vi "main.vi"() -> ()   [LabVIEW 2018]
uses:
  <vilib>/NI/Modbus Library/API/Wrapper/Create TCP Slave.vi
  <vilib>/NI/Modbus Library/API/Slave/Modbus Slave.lvclass
  <vilib>/NI/Modbus Library/API/Wrapper/API Main.lvlib
panel:
  in  "x+1":i32
  in  "擦除曲线":bool
  in  "PC启动信号":bool
  in  "PC就绪":bool
  out "远程/本地控制布尔":bool
  out "XY图":cluster{i32[], sgl[]}[](graph)
  in  "远程/本地控制":bool
  out "远程/本地控制标题":string="远程/本地"
  out "当前档位":string="当前档位"
  in  "档位目标内容":string
  out "PCTOUTAC的当前档位":string="PCTOUTAC的当前档位"
  out "档位目标内容远程":string
  in  "档位目标内容本地":string
  out "档位目标":string="配方编号"
  out "UTACTOPC的目标档位":string="UTACTOPC的配方编号"
  in  "中英文":string(combo)
  in  "编辑设定参数":bool
  in  "编辑配方":bool
  in  "退出":bool
  out "设置":string="设置"
  in  "PC换挡不成功":bool
  in  "PC换挡到位":bool
  in  "PC正在换挡":bool
  in  "PC急停":bool
  in  "PC学习":bool
  in  "PC故障":bool
  in  "PC运行/停机":bool
  out "PCOUTAC的DI信号":string="PCTOUTAC的DI信号"
  in  "UTAC复位到原点":bool
  in  "UTAC故障复位":bool
  in  "UTAC急停":bool
  in  "UTAC故障":bool
  in  "UTAC运行/停机":bool
  out "UTACTOPC的DO信号":string="UTACTOPC的DO信号"
  in  "设置":bool
  in  "总测试次数文本":string
  in  "动作数量文本":string
  in  "备注文本":string
  in  "样品编号文本":string
  in  "零件编号文本":string
  in  "零件名称文本":string
  in  "项目编号文本":string
  out "总测试次数":string="总测试次数"
  out "动作数量":string="动作数量"
  out "备注":string="备注"
  out "样品编号":string="样品编号"
  out "零件编号":string="零件编号"
  out "零件名称":string="零件名称"
  out "项目编号":string="项目编号"
  out "项目信息":string="项目信息"
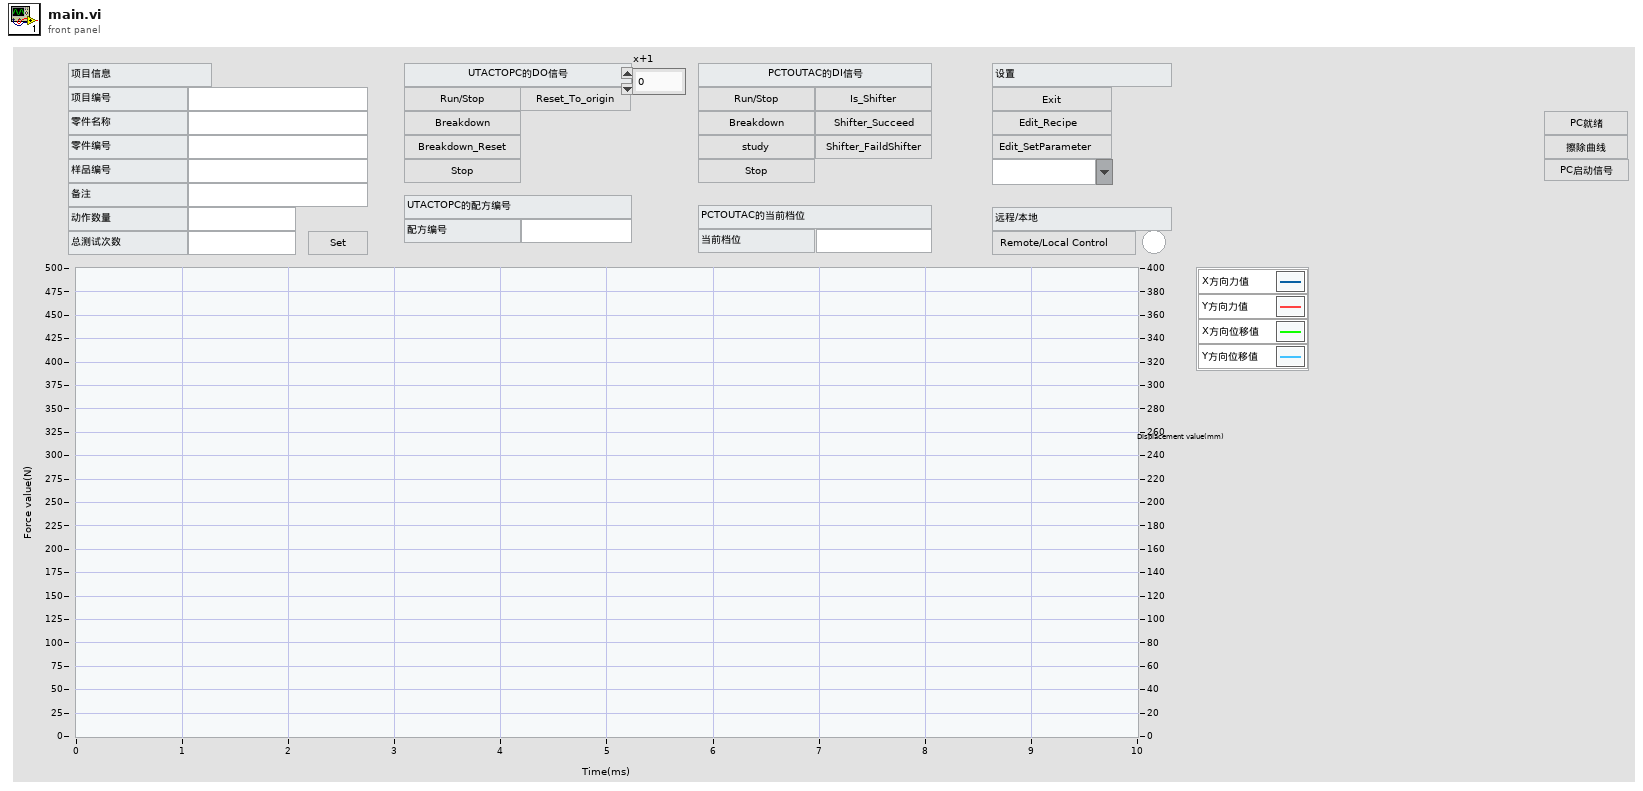
[diagram p1: front panel]
types:
  T1 = cluster{"主站IP":u32, "组号":u8, "帧号":u16, "时间戳":u64}
  T2 = cluster{"X方向力值":sgl, "Y方向力值":sgl, "X方向位移值":sgl, "Y方向位移值":sgl}
  T3 = cluster{"挡位N1所在序号":sgl, "挡位1所在序号":sgl, "挡位N1所在序号":sgl, "挡位2所在序号":sgl, "挡位N1所在序号":sgl, " 挡位N2所在序号":sgl, "挡位3所在序号":sgl, "挡位N2所在序号":sgl, "挡位4所在序号":sgl, " 挡位N2所在序号":sgl, "挡位N3所在序号":sgl, "挡位5所在序号":sgl, "挡位N3所在序号":sgl, "挡位6所在序号":sgl, "挡位N3所在序号":sgl, "挡位N4所在序号":sgl, " 挡位7所在序号":sgl, " 挡位N4所在序号":sgl, "挡位8所在序号":sgl, "挡位N4所在序号":sgl, " 挡位N5所在序号":sgl, "挡位9所在序号":sgl, "挡位N5所在序号":sgl, " 挡位10所在序号":sgl}
  T4 = cluster{"就绪":bool, "运行/停机":bool, "故障":bool, "学习":bool, "急停":bool, "正在换挡":bool, "换挡到位":bool, "换挡不成功":bool, "备用1":bool, "保存开始":bool, "等待下发任务":bool, "允许读取配方":bool, "开始采集数据":bool, "时间ON/OFF":bool, " 收到启动信号":bool, "结束采集信号":bool, "读配方参数ON/OFF":bool, "允许下发配方参数":bool}
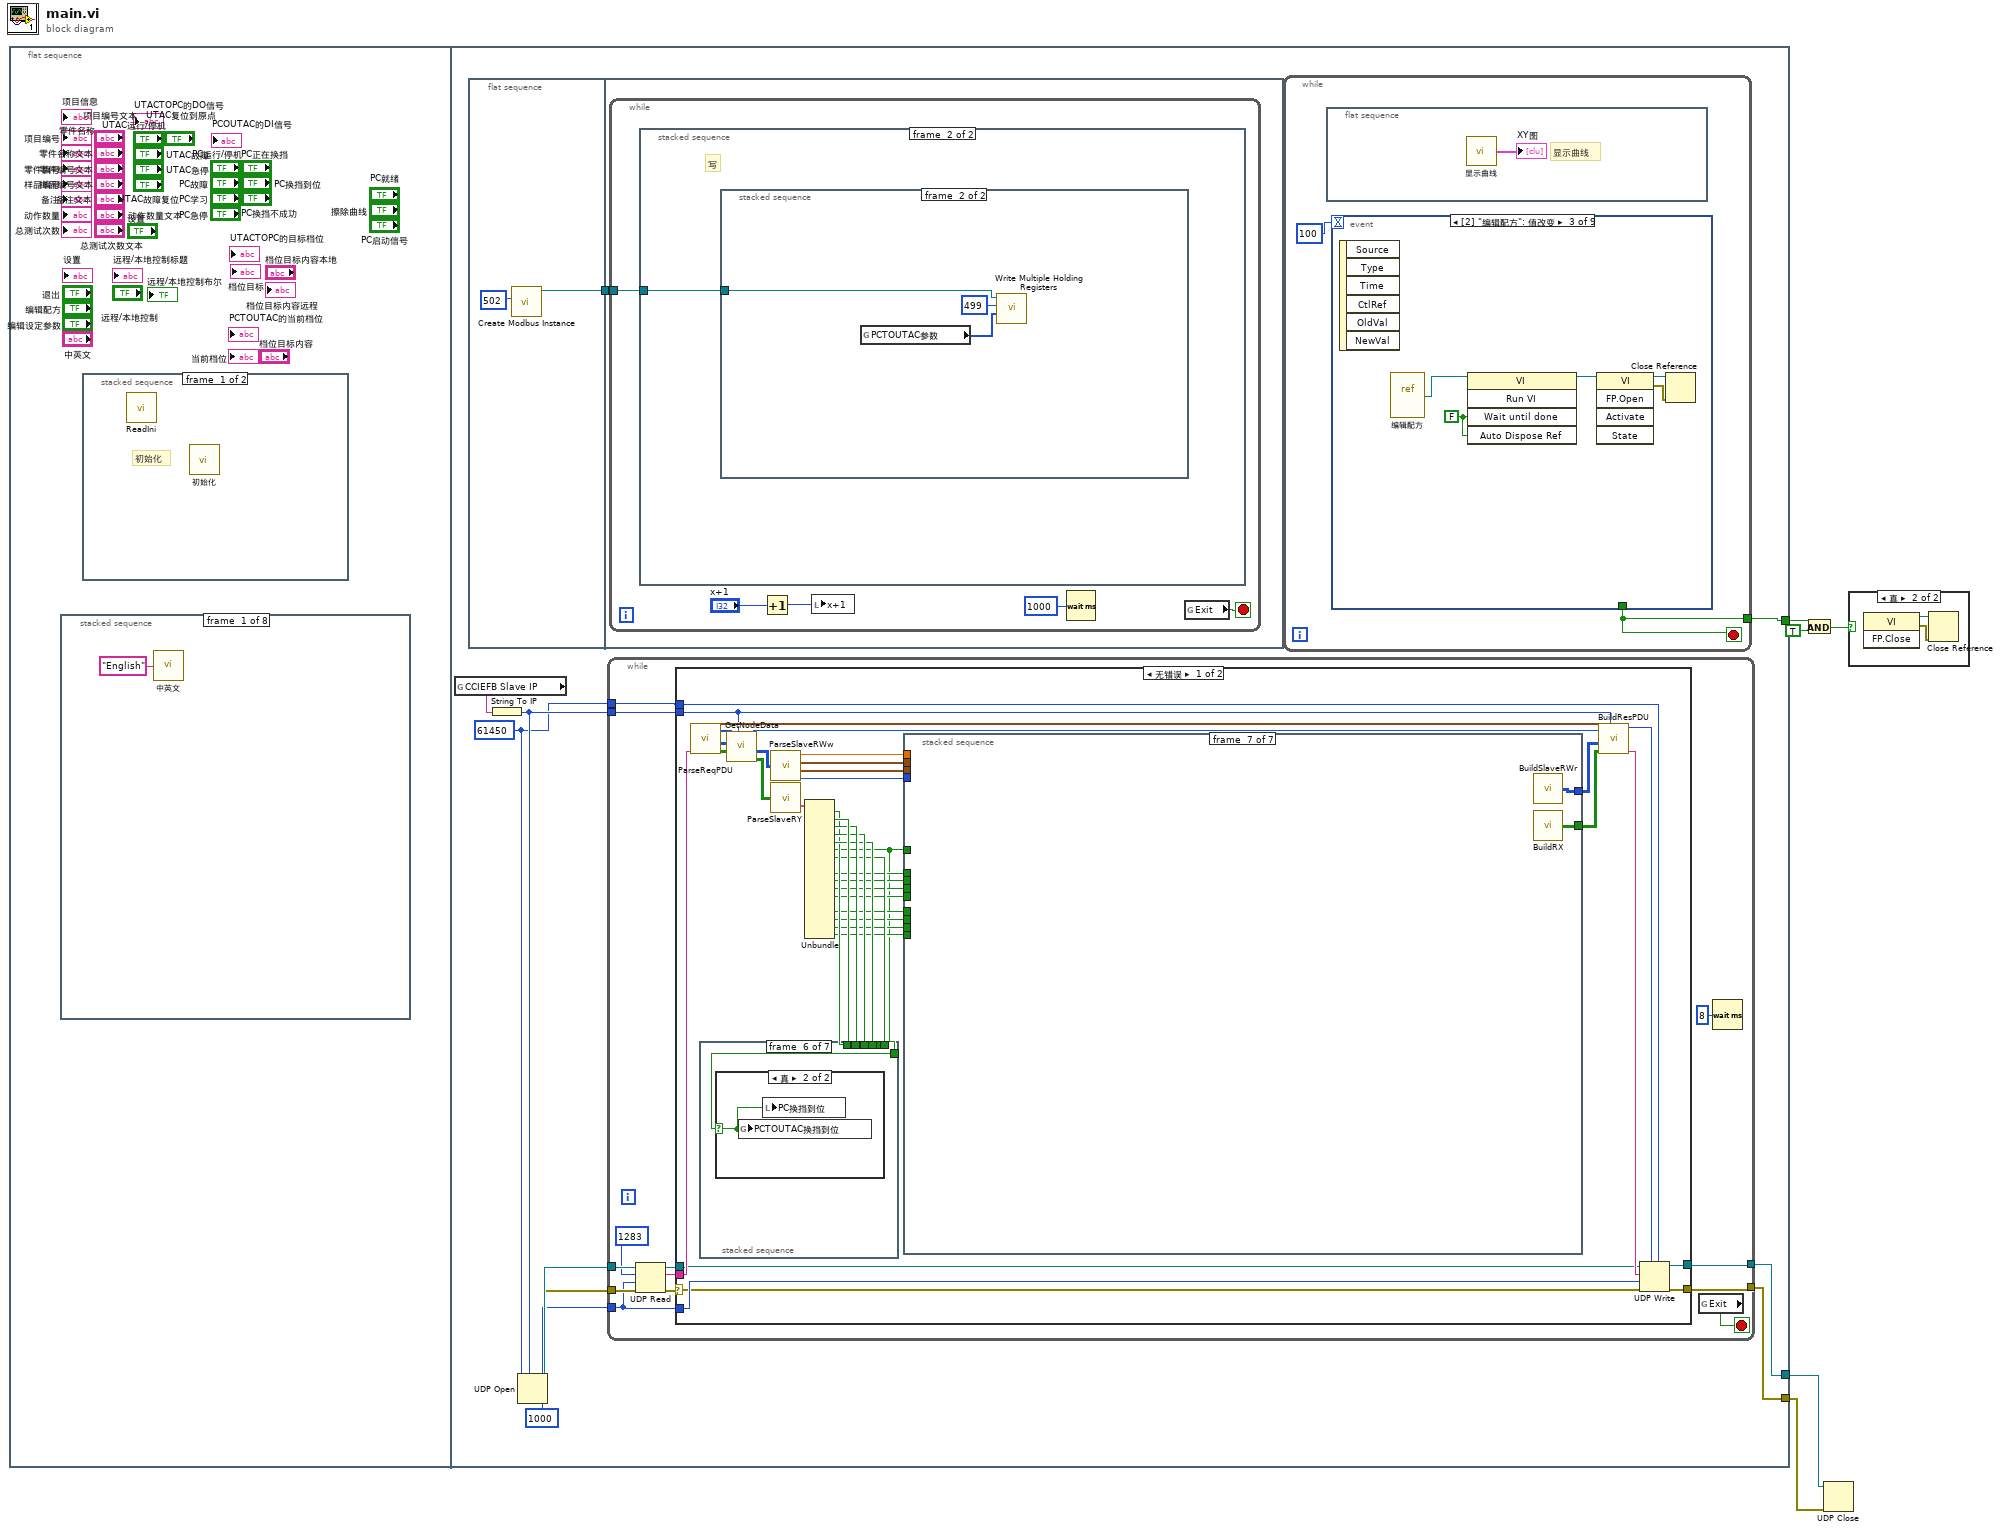
[diagram p0: block diagram]
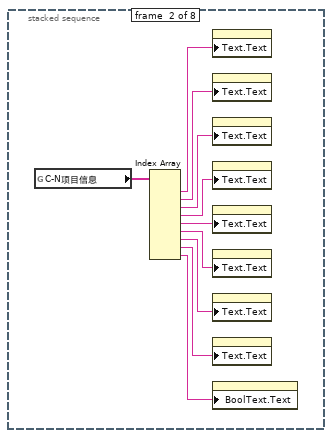
[diagram p3: hidden frame]
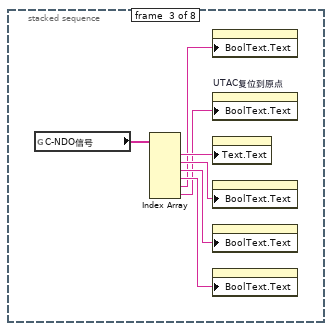
[diagram p4: hidden frame]
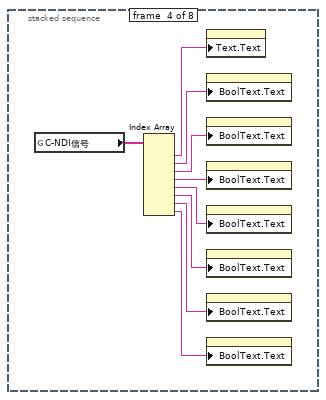
[diagram p5: hidden frame]
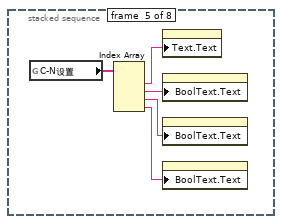
[diagram p6: hidden frame]
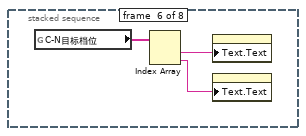
[diagram p7: hidden frame]
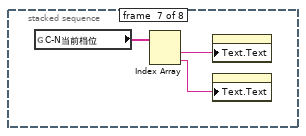
[diagram p8: hidden frame]
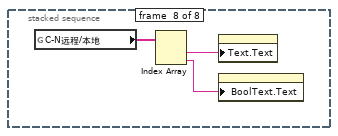
[diagram p9: hidden frame]
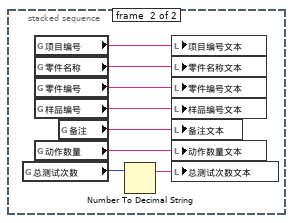
[diagram p10: hidden frame]
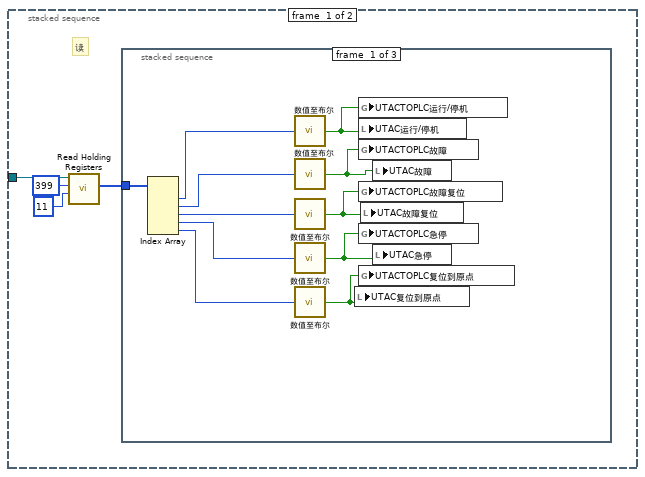
[diagram p11: hidden frame]
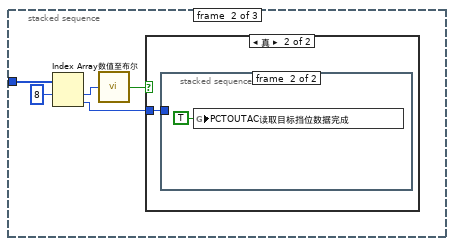
[diagram p12: hidden frame]
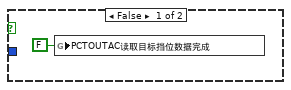
[diagram p13: hidden frame]
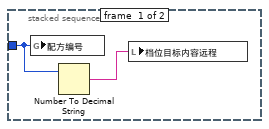
[diagram p14: hidden frame]
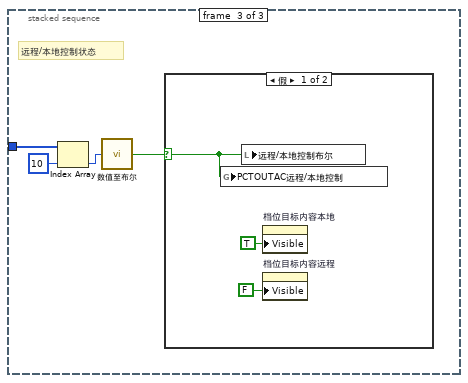
[diagram p15: hidden frame]
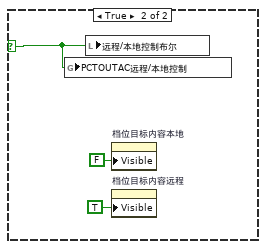
[diagram p16: hidden frame]
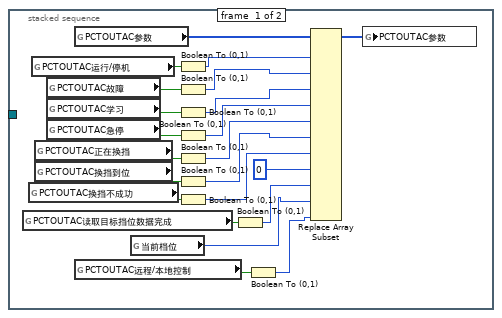
[diagram p17: hidden frame]
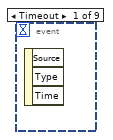
[diagram p18: hidden frame]
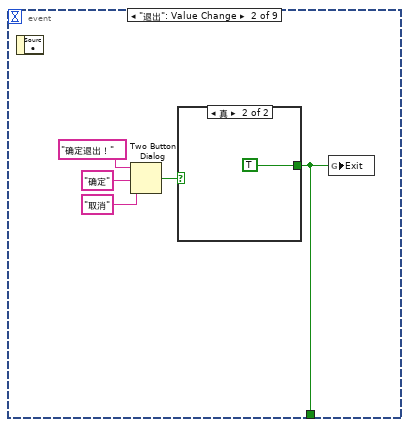
[diagram p19: hidden frame]
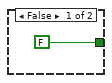
[diagram p20: hidden frame]
diagram:
  n1 = flat-sequence {
    tunnel: [w62] -> w5
    tunnel: [w61] -> w4
    tunnel: [w56] -> w3
    frame #0 {
      n2 = stacked-sequence {
        frame #0 {
          n3 = call "中英文.vi"("中英文"="English") -> ()  [unwired: 2 in]
        }
        frame #1 {
          n4 = global read "全局 1.vi" "C-N项目信息"() -> (w16:string[])
          n5 = Index Array(array=w16) -> (element #1=w15:string, element #2=w14:string, element #3=w13:string, element #4=w12:string, element #5=w11:string, element #6=w10:string, element #7=w9:string, element #8=w8:string, element #9=w7:string)  [unwired: 9 in]
          n6 = property on="项目信息" class="Str"("Text.Text"=w15) -> ()  [unwired: 2 in, 2 out]
          n7 = property on="项目编号" class="Str"("Text.Text"=w14) -> ()  [unwired: 2 in, 2 out]
          n8 = property on="零件名称" class="Str"("Text.Text"=w13) -> ()  [unwired: 2 in, 2 out]
          n9 = property on="零件编号" class="Str"("Text.Text"=w12) -> ()  [unwired: 2 in, 2 out]
          n10 = property on="样品编号" class="Str"("Text.Text"=w11) -> ()  [unwired: 2 in, 2 out]
          n11 = property on="备注" class="Str"("Text.Text"=w10) -> ()  [unwired: 2 in, 2 out]
          n12 = property on="动作数量" class="Str"("Text.Text"=w9) -> ()  [unwired: 2 in, 2 out]
          n13 = property on="总测试次数" class="Str"("Text.Text"=w8) -> ()  [unwired: 2 in, 2 out]
          n14 = property on="设置" class="Bool"("BoolText.Text"=w7) -> ()  [unwired: 2 in, 2 out]
        }
        frame #2 {
          n15 = global read "全局 1.vi" "C-NDO信号"() -> (w23:string[])
          n16 = Index Array(array=w23) -> (element #1=w22:string, element #2=w21:string, element #3=w20:string, element #4=w19:string, element #5=w18:string, element #6=w17:string)  [unwired: 6 in]
          n17 = property on="UTAC急停" class="Bool (严格)"("BoolText.Text"=w18) -> ()  [unwired: 2 in, 2 out]
          n18 = property on="UTAC复位到原点" class="Bool (严格)"("BoolText.Text"=w17) -> ()  [unwired: 2 in, 2 out]
          n19 = property on="UTACTOPC的DO信号" class="Str"("Text.Text"=w22) -> ()  [unwired: 2 in, 2 out]
          n20 = property on="UTAC运行/停机" class="Bool (严格)"("BoolText.Text"=w21) -> ()  [unwired: 2 in, 2 out]
          n21 = property on="UTAC故障" class="Bool (严格)"("BoolText.Text"=w20) -> ()  [unwired: 2 in, 2 out]
          n22 = property on="UTAC故障复位" class="Bool (严格)"("BoolText.Text"=w19) -> ()  [unwired: 2 in, 2 out]
        }
        frame #3 {
          n23 = global read "全局 1.vi" "C-NDI信号"() -> (w32:string[])
          n24 = Index Array(array=w32) -> (element #1=w31:string, element #2=w30:string, element #3=w29:string, element #4=w28:string, element #5=w27:string, element #6=w26:string, element #7=w25:string, element #8=w24:string)  [unwired: 8 in]
          n25 = property on="PCOUTAC的DI信号" class="Str"("Text.Text"=w31) -> ()  [unwired: 2 in, 2 out]
          n26 = property on="PC运行/停机" class="Bool (严格)"("BoolText.Text"=w30) -> ()  [unwired: 2 in, 2 out]
          n27 = property on="PC故障" class="Bool (严格)"("BoolText.Text"=w29) -> ()  [unwired: 2 in, 2 out]
          n28 = property on="PC学习" class="Bool (严格)"("BoolText.Text"=w28) -> ()  [unwired: 2 in, 2 out]
          n29 = property on="PC急停" class="Bool (严格)"("BoolText.Text"=w27) -> ()  [unwired: 2 in, 2 out]
          n30 = property on="PC正在换挡" class="Bool (严格)"("BoolText.Text"=w26) -> ()  [unwired: 2 in, 2 out]
          n31 = property on="PC换挡到位" class="Bool (严格)"("BoolText.Text"=w25) -> ()  [unwired: 2 in, 2 out]
          n32 = property on="PC换挡不成功" class="Bool (严格)"("BoolText.Text"=w24) -> ()  [unwired: 2 in, 2 out]
        }
        frame #4 {
          n33 = global read "全局 1.vi" "C-N设置"() -> (w37:string[])
          n34 = Index Array(array=w37) -> (element #1=w36:string, element #2=w35:string, element #3=w34:string, element #4=w33:string)  [unwired: 4 in]
          n35 = property on="设置" class="Str"("Text.Text"=w36) -> ()  [unwired: 2 in, 2 out]
          n36 = property on="退出" class="Bool"("BoolText.Text"=w35) -> ()  [unwired: 2 in, 2 out]
          n37 = property on="编辑配方" class="Bool"("BoolText.Text"=w34) -> ()  [unwired: 2 in, 2 out]
          n38 = property on="编辑设定参数" class="Bool"("BoolText.Text"=w33) -> ()  [unwired: 2 in, 2 out]
        }
        frame #5 {
          n39 = global read "全局 1.vi" "C-N目标档位"() -> (w40:string[])
          n40 = Index Array(array=w40) -> (element #1=w39:string, element #2=w38:string)  [unwired: 2 in]
          n41 = property on="UTACTOPC的目标档位" class="Str"("Text.Text"=w39) -> ()  [unwired: 2 in, 2 out]
          n42 = property on="档位目标" class="Str"("Text.Text"=w38) -> ()  [unwired: 2 in, 2 out]
        }
        frame #6 {
          n43 = global read "全局 1.vi" "C-N当前档位"() -> (w43:string[])
          n44 = Index Array(array=w43) -> (element #1=w42:string, element #2=w41:string)  [unwired: 2 in]
          n45 = property on="PCTOUTAC的当前档位" class="Str"("Text.Text"=w42) -> ()  [unwired: 2 in, 2 out]
          n46 = property on="当前档位" class="Str"("Text.Text"=w41) -> ()  [unwired: 2 in, 2 out]
        }
        frame #7 {
          n47 = global read "全局 1.vi" "C-N远程/本地"() -> (w46:string[])
          n48 = Index Array(array=w46) -> (element #1=w45:string, element #2=w44:string)  [unwired: 2 in]
          n49 = property on="远程/本地控制标题" class="Str"("Text.Text"=w45) -> ()  [unwired: 2 in, 2 out]
          n50 = property on="远程/本地控制" class="Bool (严格)"("BoolText.Text"=w44) -> ()  [unwired: 2 in, 2 out]
        }
      }
      n51 = stacked-sequence {
        frame #0 {
          # "初始化"
          n52 = call "ReadIni.vi"() -> ()  [unwired: 2 in]
          n53 = call "初始化.vi"() -> ()  [unwired: 12 in]
        }
        frame #1 {
          n54 = global read "全局 1.vi" "总测试次数"() -> (w54:i16)
          n55 = global read "全局 1.vi" "项目编号"() -> (w52:string)
          n56 = global read "全局 1.vi" "零件名称"() -> (w51:string)
          n57 = global read "全局 1.vi" "零件编号"() -> (w50:string)
          n58 = global read "全局 1.vi" "样品编号"() -> (w49:string)
          n59 = global read "全局 1.vi" "动作数量"() -> (w47:string)
          n60 = global read "全局 1.vi" "备注"() -> (w48:string)
          n61 = Number To Decimal String(number=w54) -> (decimal integer string=w53:string)  [unwired: 1 in]
          n62 = local write "项目编号文本"(w52) -> ()
          n63 = local write "零件名称文本"(w51) -> ()
          n64 = local write "零件编号文本"(w50) -> ()
          n65 = local write "样品编号文本"(w49) -> ()
          n66 = local write "备注文本"(w48) -> ()
          n67 = local write "动作数量文本"(w47) -> ()
          n68 = local write "总测试次数文本"(w53) -> ()
        }
      }
    }
    frame #1 {
      w57 = u16 61450
      n69 = global read "全局 1.vi" "CCIEFB Slave IP"() -> (w60:string)
      n70 = flat-sequence {
        tunnel: [w65] -> w55
        tunnel: w55 -> [w67]
        frame #0 {
          n71 = call-poly <vilib>:"Create Modbus Instance.vi"("port (502)"=u16 502) -> ("TCP slave instance"=w65:refnum<class "Modbus Slave.lvclass">)  [unwired: 9 in, 1 out]
        }
        frame #1 {
          n72 = while {
            tunnel: w67 -> [w71]
            stop <- w72 stop-if-true
            n73 = stacked-sequence {
              tunnel: w71 -> [w73 w108]
              frame #0 {
                # "读"
                n74 = call-dynamic "Read Holding Registers.vi"("number of inputs"=u16 11, "starting address"=u16 399, "Modbus slave in"=w73) -> ("register values"=w74:u16[])  [unwired: 6 in, 2 out]
                n75 = stacked-sequence {
                  tunnel: w74 -> [w87 w92 w101]
                  frame #0 {
                    n76 = Index Array(array=w87) -> (element #1=w86:u16, element #2=w85:u16, element #3=w84:u16, element #4=w83:u16, element #5=w82:u16)  [unwired: 5 in]
                    n77 = call "数值至布尔.vi"("数值"=w86) -> ("布尔"=w81:bool)
                    n78 = call "数值至布尔.vi"("数值"=w85) -> ("布尔"=w80:bool)
                    n79 = call "数值至布尔.vi"("数值"=w84) -> ("布尔"=w79:bool)
                    n80 = call "数值至布尔.vi"("数值"=w83) -> ("布尔"=w78:bool)
                    n81 = call "数值至布尔.vi"("数值"=w82) -> ("布尔"=w77:bool)
                    n82 = local write "UTAC复位到原点"(w77) -> ()
                    n83 = global write "全局 1.vi" "UTACTOPLC运行/停机"(w81) -> ()
                    n84 = local write "UTAC运行/停机"(w81) -> ()
                    n85 = global write "全局 1.vi" "UTACTOPLC故障"(w80) -> ()
                    n86 = global write "全局 1.vi" "UTACTOPLC故障复位"(w79) -> ()
                    n87 = global write "全局 1.vi" "UTACTOPLC急停"(w78) -> ()
                    n88 = global write "全局 1.vi" "UTACTOPLC复位到原点"(w77) -> ()
                    n89 = local write "UTAC故障复位"(w79) -> ()
                    n90 = local write "UTAC故障"(w80) -> ()
                    n91 = local write "UTAC急停"(w78) -> ()
                  }
                  frame #1 {
                    n92 = Index Array(array=w92, index #1=8 ("索引")) -> (element #1=w90:u16, element #2=w88:u16)  [unwired: 1 in]
                    n93 = call "数值至布尔.vi"("数值"=w90) -> ("布尔"=w89:bool)
                    n94 = case shown="真" w89 {
                      tunnel: w88 -> [_ w94]
                      frame False {
                        n95 = global write "全局 1.vi" "PCTOUTAC读取目标挡位数据完成"(FALSE ("PCTOUTAC读取目标挡位数据完成")) -> ()
                      }
                      frame True {
                        n96 = stacked-sequence {
                          tunnel: w94 -> [w96 _]
                          frame #0 {
                            n97 = global write "全局 1.vi" "配方编号"(w96) -> ()
                            n98 = Number To Decimal String(number=w96) -> (decimal integer string=w95:string)  [unwired: 1 in]
                            n99 = local write "档位目标内容远程"(w95) -> ()
                          }
                          frame #1 {
                            n100 = global write "全局 1.vi" "PCTOUTAC读取目标挡位数据完成"(TRUE ("PCTOUTAC读取目标挡位数据完成")) -> ()
                          }
                        }
                      }
                    }
                  }
                  frame #2 {
                    # "远程/本地控制状态"
                    n101 = Index Array(array=w101, index=10 ("索引")) -> (element=w99:u16)
                    n102 = call "数值至布尔.vi"("数值"=w99) -> ("布尔"=w98:bool)
                    n103 = case shown="假" w98 {
                      selector: w98 -> [w104 w107]
                      frame False {
                        n104 = global write "全局 1.vi" "PCTOUTAC远程/本地控制"(w104) -> ()
                        n105 = local write "远程/本地控制布尔"(w104) -> ()
                        n106 = property on="档位目标内容本地" class="Str"("Visible"=TRUE ("可见")) -> ()  [unwired: 2 in, 2 out]
                        n107 = property on="档位目标内容远程" class="Str"("Visible"=FALSE ("可见")) -> ()  [unwired: 2 in, 2 out]
                      }
                      frame True {
                        n108 = global write "全局 1.vi" "PCTOUTAC远程/本地控制"(w107) -> ()
                        n109 = local write "远程/本地控制布尔"(w107) -> ()
                        n110 = property on="档位目标内容本地" class="Str"("Visible"=FALSE ("可见")) -> ()  [unwired: 2 in, 2 out]
                        n111 = property on="档位目标内容远程" class="Str"("Visible"=TRUE ("可见")) -> ()  [unwired: 2 in, 2 out]
                      }
                    }
                  }
                }
              }
              frame #1 {
                # "写"
                n112 = stacked-sequence {
                  tunnel: w108 -> [_ w133]
                  frame #0 {
                    n113 = global read "全局 1.vi" "PCTOUTAC读取目标挡位数据完成"() -> (w113:bool)
                    n114 = global read "全局 1.vi" "PCTOUTAC换挡不成功"() -> (w124:bool)
                    n115 = global read "全局 1.vi" "PCTOUTAC运行/停机"() -> (w130:bool)
                    n116 = global read "全局 1.vi" "PCTOUTAC正在换挡"() -> (w126:bool)
                    n117 = global read "全局 1.vi" "PCTOUTAC换挡到位"() -> (w125:bool)
                    n118 = global read "全局 1.vi" "PCTOUTAC故障"() -> (w129:bool)
                    n119 = global read "全局 1.vi" "PCTOUTAC学习"() -> (w128:bool)
                    n120 = global read "全局 1.vi" "PCTOUTAC急停"() -> (w127:bool)
                    n121 = global read "全局 1.vi" "PCTOUTAC参数"() -> (w123:i16[])
                    n122 = global read "全局 1.vi" "PCTOUTAC远程/本地控制"() -> (w110:bool)
                    n123 = global read "全局 1.vi" "当前档位"() -> (w111:u16)
                    n124 = Boolean To (0,1)(Boolean=w130) -> (0, 1=w122:i16)
                    n125 = Boolean To (0,1)(Boolean=w129) -> (0, 1=w120:i16)
                    n126 = Boolean To (0,1)(Boolean=w128) -> (0, 1=w119:i16)
                    n127 = Boolean To (0,1)(Boolean=w127) -> (0, 1=w118:i16)
                    n128 = Boolean To (0,1)(Boolean=w126) -> (0, 1=w117:i16)
                    n129 = Boolean To (0,1)(Boolean=w125) -> (0, 1=w116:i16)
                    n130 = Boolean To (0,1)(Boolean=w124) -> (0, 1=w115:i16)
                    n131 = Boolean To (0,1)(Boolean=w113) -> (0, 1=w112:i16)
                    n132 = Boolean To (0,1)(Boolean=w110) -> (0, 1=w109:i16)
                    n133 = Replace Array Subset(array=w123, new element #1=w122, new element #2=w120, new element #3=w119, new element #4=w118, new element #5=w117, new element #6=w116, new element #7=w115, new element #8=i16 0 ("新元素/子数组"), new element #9=w112, new element #10=w111, new element #11=w109) -> (w121:i16[])  [unwired: 11 in]
                    n134 = global write "全局 1.vi" "PCTOUTAC参数"(w121) -> ()
                  }
                  frame #1 {
                    n135 = global read "全局 1.vi" "PCTOUTAC参数"() -> (w131:i16[])
                    n136 = call-dynamic "Write Multiple Holding Registers.vi"("registers to write"=w131, "starting address"=u16 499, "Modbus slave in"=w133) -> ()  [unwired: 7 in, 2 out]
                  }
                }
              }
            }
            n137 = Increment(x="x+1") -> (x+1=w68:i32)
            n138 = local write "x+1"(w68) -> ()
            n139 = Wait (ms)(milliseconds to wait=u32 1000 ("等待时间（毫秒）")) -> ()  [unwired: 1 out]
            n140 = global read "全局 1.vi" "Exit"() -> (w72:bool)
          }
        }
      }
      n141 = String To IP(1:w60) -> (0:w58:u32)
      n142 = UDP Open(7:w58, 11:w57) -> (port=w64:refnum<k16>, 0:w63:errorcluster)  [unwired: 3 in, 1 out]
      n143 = while {
        tunnel: w64 -> [w220]
        tunnel: w63 -> [w219]
        tunnel: [w212] -> w62
        tunnel: [w211] -> w61
        tunnel: 1000 -> [w210]
        tunnel: w58 -> [w213]
        tunnel: w57 -> [w209]
        stop <- w218 stop-if-true
        n144 = UDP Read(connection ID=w220, max size (548)=1283 ("最大值(548)"), timeout ms (25000)=w210, 8:w219) -> (data out=w215:string, error out=w216:errorcluster, 3:w214:refnum<k16>)  [unwired: 2 out]
        n145 = case shown="无错误" w216 {
          selector: w216 -> [w247 w364]
          tunnel: w215 -> [w259 _]
          tunnel: w214 -> [w249 w362]
          tunnel: [w252 w363] -> w211
          tunnel: [w251 w362] -> w212
          tunnel: w213 -> [w244 _]
          tunnel: w210 -> [w248 _]
          tunnel: w209 -> [w243 _]
          frame No Error {
            n146 = call "ParseReqPDU.vi"("数据in"=w259) -> ("All RY"=w256:bool[][], "All RWw"=w257:u16[][], "从站IP组"=w258:u32[], "主站信息"=w253:T1)  [unwired: 7 in]
            n147 = call "GetNodeData.vi"("指定从站IP"=w244, "All RY in"=w256, "All RWw in"=w257, "从站IP组"=w258) -> ("Node RY"=w254:bool[][], "Node RWw"=w255:u16[][], "占用站数"=w245:i32)  [unwired: 5 in]
            n148 = call "ParseSlaveRWw.vi"("Node RWw"=w255) -> ("当前档位"=w240:sgl, "PLC采集值"=w239:T2, "PLC档位序号"=w238:T3, "行号"=w237:i32)
            n149 = call "ParseSlaveRY.vi"("RY"=w254) -> ("PLC状态"=w236:T4)  [unwired: 1 in]
            n150 = Unbundle(w236) -> ("运行/停机"=w231:bool, "故障"=w235:bool, "学习"=w234:bool, "急停"=w233:bool, "正在换挡"=w232:bool, "换挡到位"=w221:bool, "换挡不成功"=w230:bool, "保存开始"=w229:bool, "等待下发任务"=w228:bool, "允许读取配方"=w222:bool, "开始采集数据"=w227:bool, "收到启动信号"=w225:bool, "结束采集信号"=w226:bool, "读配方参数ON/OFF"=w224:bool, "允许下发配方参数"=w223:bool)  [unwired: 3 out]
            n151 = stacked-sequence {
              tunnel: w231 -> [w260 _ _ _ _ _ _]
              tunnel: w235 -> [_ w262 _ _ _ _ _]
              tunnel: w234 -> [_ _ w264 _ _ _ _]
              tunnel: w233 -> [_ _ _ w266 _ _ _]
              tunnel: w232 -> [_ _ _ _ w268 _ w272]
              tunnel: w221 -> [_ _ _ _ _ w270 _]
              tunnel: w230 -> [_ _ _ _ _ _ _]
              frame #0 {
                n152 = case shown="真" w260 {
                  selector: w260 -> [_ w261]
                  frame False {
                  }
                  frame True {
                    n153 = global write "全局 1.vi" "PCTOUTAC运行/停机"(w261) -> ()
                    n154 = local write "PC运行/停机"(w261) -> ()
                  }
                }
              }
              frame #1 {
                n155 = case shown="真" w262 {
                  selector: w262 -> [_ w263]
                  frame False {
                  }
                  frame True {
                    n156 = global write "全局 1.vi" "PCTOUTAC故障"(w263) -> ()
                    n157 = local write "PC故障"(w263) -> ()
                  }
                }
              }
              frame #2 {
                n158 = case shown="真" w264 {
                  selector: w264 -> [_ w265]
                  frame False {
                  }
                  frame True {
                    n159 = global write "全局 1.vi" "PCTOUTAC学习"(w265) -> ()
                    n160 = local write "PC学习"(w265) -> ()
                  }
                }
              }
              frame #3 {
                n161 = case shown="真" w266 {
                  selector: w266 -> [_ w267]
                  frame False {
                  }
                  frame True {
                    n162 = global write "全局 1.vi" "PCTOUTAC急停"(w267) -> ()
                    n163 = local write "PC急停"(w267) -> ()
                  }
                }
              }
              frame #4 {
                n164 = case shown="真" w268 {
                  selector: w268 -> [_ w269]
                  frame False {
                  }
                  frame True {
                    n165 = global write "全局 1.vi" "PCTOUTAC正在换挡"(w269) -> ()
                    n166 = local write "PC正在换挡"(w269) -> ()
                  }
                }
              }
              frame #5 {
                n167 = case shown="真" w270 {
                  selector: w270 -> [_ w271]
                  frame False {
                  }
                  frame True {
                    n168 = global write "全局 1.vi" "PCTOUTAC换挡到位"(w271) -> ()
                    n169 = local write "PC换挡到位"(w271) -> ()
                  }
                }
              }
              frame #6 {
                n170 = case shown="真" w272 {
                  selector: w272 -> [_ w273]
                  frame False {
                  }
                  frame True {
                    n171 = global write "全局 1.vi" "PCTOUTAC正在换挡"(w273) -> ()
                    n172 = local write "PC换挡不成功"(w273) -> ()
                  }
                }
              }
            }
            n173 = stacked-sequence {
              tunnel: [_ _ _ _ _ _ w361] -> w242
              tunnel: [_ _ _ _ _ _ w360] -> w241
              tunnel: w240 -> [_ _ _ _ w322 _ _]
              tunnel: w239 -> [_ _ _ _ w323 _ _]
              tunnel: w238 -> [_ _ _ w305 _ _ _]
              tunnel: w237 -> [_ _ _ _ _ w342 _]
              tunnel: w229 -> [w275 w293 _ _ _ _ _]
              tunnel: w228 -> [w274 _ w296 _ _ _ _]
              tunnel: w222 -> [w279 _ _ w306 _ _ _]
              tunnel: w227 -> [_ _ _ _ w325 _ _]
              tunnel: w226 -> [_ _ _ _ _ _ _]
              tunnel: w225 -> [w278 _ _ _ w324 _ _]
              tunnel: w224 -> [w276 _ _ _ _ w344 _]
              tunnel: w223 -> [w277 _ _ _ _ w343 _]
              tunnel: w221 -> [_ _ _ _ w321 _ _]
              frame #0 {
                # "收到启动信号"
                n174 = stacked-sequence {
                  tunnel: w279 -> [_ _ w284 _ _ _]
                  tunnel: w278 -> [_ _ _ w286 _ _]
                  tunnel: w277 -> [_ _ _ _ w288 _]
                  tunnel: w276 -> [_ _ _ _ _ w290]
                  tunnel: w275 -> [w280 _ _ _ _ _]
                  tunnel: w274 -> [_ w282 _ _ _ _]
                  frame #0 {
                    n175 = case shown="假" w280 {
                      frame False {
                        n176 = global write "全局 1.vi" "PCTOPLC保存完成"(FALSE ("PCTOPLC保存完成")) -> ()
                      }
                      frame True {
                      }
                    }
                  }
                  frame #1 {
                    n177 = case shown="假" w282 {
                      frame False {
                        n178 = global write "全局 1.vi" "PCTOPLC下发任务完成"(FALSE ("PCTOPLC保存完成")) -> ()
                      }
                      frame True {
                      }
                    }
                  }
                  frame #2 {
                    n179 = case shown="假" w284 {
                      frame False {
                        n180 = global write "全局 1.vi" "PCTOPLC读取配方完成"(FALSE ("PCTOUTAC换挡到位")) -> ()
                      }
                      frame True {
                      }
                    }
                  }
                  frame #3 {
                    n181 = case shown="假" w286 {
                      frame False {
                        n182 = global write "全局 1.vi" "PCTOPLC发送启动信号"(FALSE ("PCTOUTAC换挡到位")) -> ()
                      }
                      frame True {
                      }
                    }
                  }
                  frame #4 {
                    n183 = case shown="假" w288 {
                      frame False {
                        n184 = global write "全局 1.vi" "PCTOPLC下发配方参数完成"(FALSE ("PCTOPLC下发配方参数完成")) -> ()
                      }
                      frame True {
                      }
                    }
                  }
                  frame #5 {
                    n185 = case shown="假" w290 {
                      frame False {
                        n186 = global write "全局 1.vi" "PCTOPLC读配方结束"(FALSE ("PCTOPLC下发配方参数完成")) -> ()
                      }
                      frame True {
                      }
                    }
                  }
                }
              }
              frame #1 {
                # "保存"
                n187 = call "BuildEdgePulse.vi"("输入"=w293) -> ("上升沿"=w292:bool)  [unwired: 2 in, 2 out]
                n188 = case shown="真" w292 {
                  frame False {
                  }
                  frame True {
                    n189 = stacked-sequence {
                      frame #0 {
                        n190 = call "保存模版.vi"() -> ()  [unwired: 12 in]
                      }
                      frame #1 {
                        n191 = global write "全局 1.vi" "PCTOPLC保存完成"(TRUE ("PCTOPLC保存完成")) -> ()
                      }
                    }
                  }
                }
              }
              frame #2 {
                # "等待下发任务"
                n192 = call "BuildEdgePulse.vi"("输入"=w296) -> ("上升沿"=w295:bool)  [unwired: 2 in, 2 out]
                n193 = case shown="真" w295 {
                  frame False {
                  }
                  frame True {
                    n194 = stacked-sequence {
                      frame #0 {
                        n195 = global read "全局 1.vi" "配方编号"() -> (w301:u16)
                        n196 = call "配方.vi"() -> ("起始行号"=w303:string[], "终止行号"=w302:string[])  [unwired: 1 in]
                        n197 = Index Array(array=w303, index=w301) -> (element=w300:string)
                        n198 = Index Array(array=w302, index=w301) -> (element=w299:string)
                        n199 = Decimal String To Number(string=w300) -> (number=w298:i32)  [unwired: 2 in, 1 out]
                        n200 = Decimal String To Number(string=w299) -> (number=w297:i32)  [unwired: 2 in, 1 out]
                        n201 = global write "全局 1.vi" "起始序号"(w298) -> ()
                        n202 = global write "全局 1.vi" "终止序号"(w297) -> ()
                      }
                      frame #1 {
                        n203 = global write "全局 1.vi" "PCTOPLC下发任务完成"(TRUE ("PCTOPLC下发任务完成")) -> ()
                      }
                    }
                  }
                }
              }
              frame #3 {
                # "允许读取配方：从PLC读取档位所在行号写入plcrecipe.csv"
                n204 = call "BuildEdgePulse.vi"("输入"=w306) -> ("上升沿"=w307:bool)  [unwired: 2 in, 2 out]
                n205 = case shown="真" w307 {
                  tunnel: w305 -> [_ w308]
                  frame False {
                  }
                  frame True {
                    n206 = stacked-sequence {
                      tunnel: w308 -> [w317 _]
                      frame #0 {
                        w313 = string[] ["N", "R", "N", "1", "2"]
                        n207 = for {
                          tunnel: w313 -> [_] mode=indexing
                          tunnel: [w318] -> w315 mode=indexing
                          i -> [w319]
                          n208 = Increment(x=w319) -> (x+1=w318:i32)
                        }
                        n209 = Cluster To Array(cluster=w317) -> (array=w316:sgl[])
                        n210 = Number To Decimal String(number=w316) -> (decimal integer string=w312:string[])  [unwired: 1 in]
                        n211 = Number To Decimal String(number=w315) -> (decimal integer string=w314:string[])  [unwired: 1 in]
                        n212 = Build Array(w314, w313, w312) -> (w311:string[][])
                        n213 = Transpose 2D Array(2D array=w311) -> (transposed array=w310:string[][])
                        n214 = call "WriteCsv.vi"("相对路径"="plcrecipe.csv", "2D data"=w310) -> ()  [unwired: 2 in, 1 out]
                      }
                      frame #1 {
                        n215 = global write "全局 1.vi" "PCTOPLC读取配方完成"(TRUE ("PCTOPLC读取配方完成")) -> ()
                      }
                    }
                  }
                }
              }
              frame #4 {
                n216 = case shown="真" w325 {
                  selector: w325 -> [_ w329]
                  tunnel: w324 -> [_ w328]
                  tunnel: w323 -> [_ w330]
                  tunnel: w322 -> [_ w327]
                  tunnel: w321 -> [_ w326]
                  frame False {
                  }
                  frame True {
                    n217 = stacked-sequence {
                      tunnel: w330 -> [_ w336]
                      tunnel: w329 -> [w332 _]
                      tunnel: w328 -> [_ w335]
                      tunnel: w327 -> [_ w334]
                      tunnel: w326 -> [_ w333]
                      frame #0 {
                        n218 = call "BuildEdgePulse.vi"("输入"=w332) -> ("上升沿"=w331:bool)  [unwired: 2 in, 2 out]
                        n219 = case shown="真" w331 {
                          frame False {
                          }
                          frame True {
                            n220 = call "初始化.vi"() -> ()  [unwired: 12 in]
                          }
                        }
                      }
                      frame #1 {
                        n221 = case shown="假" w335 {
                          tunnel: w336 -> [w339 _]
                          tunnel: w334 -> [w337 _]
                          tunnel: w333 -> [w338 _]
                          frame False {
                            # "开始采集"
                            n222 = call "转换数组簇.vi"("PLC采集值"=w339) -> ()  [unwired: 2 in]
                            n223 = case shown="真" w338 {
                              tunnel: w337 -> [_ w340]
                              frame False {
                              }
                              frame True {
                                # "换档到位"
                                n224 = global write "全局 1.vi" "当前档位"(w340) -> ()
                                n225 = Number To Decimal String(number=w340) -> (decimal integer string=w341:string)  [unwired: 1 in]
                                n226 = property on="档位目标内容" class="Str"("Value"=w341) -> ()  [unwired: 2 in, 2 out]
                              }
                            }
                          }
                          frame True {
                            # "结束采集"
                          }
                        }
                      }
                    }
                  }
                }
              }
              frame #5 {
                # "读取设定参数：将UTAC设定参数写入到PLC"
                n227 = case shown="真" w344 {
                  tunnel: w343 -> [_ w347]
                  tunnel: w342 -> [_ w345]
                  frame False {
                  }
                  frame True {
                    n228 = call "BuildEdgePulse.vi"("输入"=w347) -> ("上升沿"=w346:bool)  [unwired: 2 in, 2 out]
                    n229 = case shown="真" w346 {
                      tunnel: w345 -> [_ w348]
                      frame False {
                      }
                      frame True {
                        n230 = stacked-sequence {
                          tunnel: w348 -> [w350 _]
                          frame #0 {
                            n231 = Decrement(x=w350) -> (x-1=w349:i32)
                            n232 = call "ReadCsv.vi"("相对路径"="settingparameter.csv") -> ("all rows"=w354:string[][])  [unwired: 1 in]
                            n233 = Index Array(array=w354, index (row)=w349) -> (element=w351:string[])  [unwired: 1 in]
                            n234 = Array Size(array=w351) -> (size(s)=w352:i32)
                            n235 = Less Or Equal?(x=w350, y=w352) -> (x <= y?=w353:bool)
                            n236 = case shown="真" w353 {
                              tunnel: w351 -> [_ w357]
                              frame False {
                                n237 = global write "全局 1.vi" "PCTOPLC读配方结束"(TRUE ("PCTOPLC下发配方参数完成")) -> ()
                              }
                              frame True {
                                n238 = Decimal String To Number(string=w357) -> (number=w358:i32[])  [unwired: 2 in, 1 out]
                                n239 = global write "全局 1.vi" "UTAC设定参数"(w358) -> ()
                              }
                            }
                          }
                          frame #1 {
                            n240 = global write "全局 1.vi" "PCTOPLC下发配方参数完成"(TRUE ("PCTOPLC下发配方参数完成")) -> ()
                          }
                        }
                      }
                    }
                  }
                }
              }
              frame #6 {
                n241 = call "BuildSlaveRWr.vi"() -> ("RWr"=w361:i16[][])  [unwired: 1 in]
                n242 = call "BuildRX.vi"() -> ("RX"=w360:bool[][])  [unwired: 6 in]
              }
            }
            n243 = call "BuildResPDU.vi"("从站IP"=w244, "Node RX"=w241, "Node RWr"=w242, "占用站数"=w245, "主站信息"=w253) -> ("输出字符串"=w250:string, "主站IP"=w246:u32)  [unwired: 5 in]
            n244 = UDP Write(address=w246, port or service name=w243, connection ID=w249, data in=w250, 8:w247, 9:w248) -> (error out=w252:errorcluster, 3:w251:refnum<k16>)
          }
          frame Error {
            n245 = Unbundle By Name(w364) -> ("code"=w365:i32)
            n246 = case shown="默认" w365 {
              tunnel: w364 -> [w366 _]
              tunnel: [w366 errorcluster {"status"=FALSE, "code"=0, "source"=""} ("error IO")] -> w363
              frame Default {
              }
              frame 56 {
              }
            }
          }
        }
        n247 = global read "全局 1.vi" "Exit"() -> (w218:bool)
        n248 = Wait (ms)(milliseconds to wait=u32 8 ("等待时间（毫秒）")) -> ()  [unwired: 1 out]
      }
      n249 = while {
        tunnel: [w134] -> w56
        stop <- w134 stop-if-true
        n250 = flat-sequence {
          frame #0 {
            # "显示曲线"
            n251 = call "显示曲线.vi"() -> ("曲线数组"=→"XY图":cluster{i32[], sgl[]}[])  [unwired: 2 in]
          }
        }
        n252 = event shown="[2] \"编辑配方\": 值改变" {
          selector: _ -> [_ _ _ _ _ _ _ _ _]
          dyn-events: _ -> [_ _ _ _ _ _ _ _ _]
          timeout: 100 -> [_ _ _ _ _ _ _ _ _]
          tunnel: [_ w137 _ _ _ _ _ _ _] -> w134
          event Timeout {
            n253 = event-data() -> ()  [unwired: 1 in, 3 out]
          }
          event "退出": Value Change {
            n254 = event-data() -> ()  [unwired: 1 in, 1 out]
            n255 = Two Button Dialog(message="确定退出！" ("消息"), 1:"取消" ("F按钮名称（“取消”）"), 2:"确定" ("T按钮名称（“确定”）")) -> (T button?=w138:bool)
            n256 = case shown="真" w138 {
              tunnel: [FALSE TRUE] -> w137
              frame False {
              }
              frame True {
              }
            }
            n257 = global write "全局 1.vi" "Exit"(w137) -> ()
          }
          event "编辑配方": Value Change {
            w147 = FALSE ("结束前等待")
            n258 = event-data() -> ()  [unwired: 1 in, 6 out]
            n259 = vi-ref "编辑配方.vi"() -> (w148:refnum<vi>)
            n260 = invoke class="VI" method="Run VI"(reference=w148, "Wait until done"=w147, "Auto Dispose Ref"=w147) -> (reference out=w146:refnum<vi>)  [unwired: 2 in, 4 out]
            n261 = invoke class="VI" method="FP.Open"(reference=w146) -> (reference out=w145:refnum<vi>, error out=w144:errorcluster)  [unwired: 4 in, 3 out]
            n262 = Close Reference(reference=w145, error in (no error)=w144) -> ()  [unwired: 1 out]
          }
          event "设置": Value Change {
            n263 = event-data() -> ()  [unwired: 1 in, 1 out]
            n264 = local read "总测试次数文本"() -> (w150:string)
            n265 = local read "项目编号文本"() -> (w156:string)
            n266 = local read "零件名称文本"() -> (w155:string)
            n267 = local read "零件编号文本"() -> (w154:string)
            n268 = local read "样品编号文本"() -> (w153:string)
            n269 = local read "动作数量文本"() -> (w151:string)
            n270 = local read "备注文本"() -> (w152:string)
            n271 = Decimal String To Number(string=w150) -> (number=w149:i32)  [unwired: 2 in, 1 out]
            n272 = global write "全局 1.vi" "项目编号"(w156) -> ()
            n273 = global write "全局 1.vi" "零件名称"(w155) -> ()
            n274 = global write "全局 1.vi" "零件编号"(w154) -> ()
            n275 = global write "全局 1.vi" "样品编号"(w153) -> ()
            n276 = global write "全局 1.vi" "备注"(w152) -> ()
            n277 = global write "全局 1.vi" "动作数量"(w151) -> ()
            n278 = global write "全局 1.vi" "总测试次数"(w149) -> ()
            n279 = call "WriteIni.vi"() -> ()  [unwired: 2 in]
          }
          event "档位目标内容本地": Value Change {
            n280 = event-data() -> ("NewVal"=w158:string)  [unwired: 1 in]
            n281 = Decimal String To Number(string=w158) -> (number=w157:i32)  [unwired: 2 in, 1 out]
            n282 = global write "全局 1.vi" "配方编号"(w157) -> ()
          }
          event "编辑设定参数": Value Change {
            w163 = FALSE ("结束前等待")
            n283 = event-data() -> ()  [unwired: 1 in, 6 out]
            n284 = vi-ref "编辑设定参数.vi"() -> (w160:refnum<vi>)
            n285 = invoke class="VI" method="Run VI"(reference=w160, "Wait until done"=w163, "Auto Dispose Ref"=w163) -> (reference out=w162:refnum<vi>, error out=w161:errorcluster)  [unwired: 2 in, 3 out]
            n286 = invoke class="VI" method="FP.Open"(reference=w162, error in=w161) -> (reference out=w159:refnum<vi>, error out=w164:errorcluster)  [unwired: 3 in, 3 out]
            n287 = Close Reference(reference=w159, error in (no error)=w164) -> ()  [unwired: 1 out]
          }
          event "中英文": Value Change {
            n288 = event-data() -> ("NewVal"=w165:string)  [unwired: 1 in]
            n289 = stacked-sequence {
              tunnel: w165 -> [w166 _ _ _ _ _ _ _]
              frame #0 {
                n290 = call "中英文.vi"("中英文"=w166) -> ()  [unwired: 2 in]
              }
              frame #1 {
                n291 = global read "全局 1.vi" "C-N项目信息"() -> (w176:string[])
                n292 = Index Array(array=w176) -> (element #1=w175:string, element #2=w174:string, element #3=w173:string, element #4=w172:string, element #5=w171:string, element #6=w170:string, element #7=w169:string, element #8=w168:string, element #9=w167:string)  [unwired: 9 in]
                n293 = property on="项目信息" class="Str"("Text.Text"=w175) -> ()  [unwired: 2 in, 2 out]
                n294 = property on="项目编号" class="Str"("Text.Text"=w174) -> ()  [unwired: 2 in, 2 out]
                n295 = property on="零件名称" class="Str"("Text.Text"=w173) -> ()  [unwired: 2 in, 2 out]
                n296 = property on="零件编号" class="Str"("Text.Text"=w172) -> ()  [unwired: 2 in, 2 out]
                n297 = property on="样品编号" class="Str"("Text.Text"=w171) -> ()  [unwired: 2 in, 2 out]
                n298 = property on="备注" class="Str"("Text.Text"=w170) -> ()  [unwired: 2 in, 2 out]
                n299 = property on="动作数量" class="Str"("Text.Text"=w169) -> ()  [unwired: 2 in, 2 out]
                n300 = property on="总测试次数" class="Str"("Text.Text"=w168) -> ()  [unwired: 2 in, 2 out]
                n301 = property on="设置" class="Bool"("BoolText.Text"=w167) -> ()  [unwired: 2 in, 2 out]
              }
              frame #2 {
                n302 = global read "全局 1.vi" "C-NDO信号"() -> (w183:string[])
                n303 = Index Array(array=w183) -> (element #1=w182:string, element #2=w181:string, element #3=w180:string, element #4=w179:string, element #5=w178:string, element #6=w177:string)  [unwired: 6 in]
                n304 = property on="UTACTOPC的DO信号" class="Str"("Text.Text"=w182) -> ()  [unwired: 2 in, 2 out]
                n305 = property on="UTAC运行/停机" class="Bool (严格)"("BoolText.Text"=w181) -> ()  [unwired: 2 in, 2 out]
                n306 = property on="UTAC故障" class="Bool (严格)"("BoolText.Text"=w180) -> ()  [unwired: 2 in, 2 out]
                n307 = property on="UTAC故障复位" class="Bool (严格)"("BoolText.Text"=w179) -> ()  [unwired: 2 in, 2 out]
                n308 = property on="UTAC急停" class="Bool (严格)"("BoolText.Text"=w178) -> ()  [unwired: 2 in, 2 out]
                n309 = property on="UTAC复位到原点" class="Bool (严格)"("BoolText.Text"=w177) -> ()  [unwired: 2 in, 2 out]
              }
              frame #3 {
                n310 = global read "全局 1.vi" "C-NDI信号"() -> (w192:string[])
                n311 = Index Array(array=w192) -> (element #1=w191:string, element #2=w190:string, element #3=w189:string, element #4=w188:string, element #5=w187:string, element #6=w186:string, element #7=w185:string, element #8=w184:string)  [unwired: 8 in]
                n312 = property on="PCOUTAC的DI信号" class="Str"("Text.Text"=w191) -> ()  [unwired: 2 in, 2 out]
                n313 = property on="PC运行/停机" class="Bool (严格)"("BoolText.Text"=w190) -> ()  [unwired: 2 in, 2 out]
                n314 = property on="PC故障" class="Bool (严格)"("BoolText.Text"=w189) -> ()  [unwired: 2 in, 2 out]
                n315 = property on="PC学习" class="Bool (严格)"("BoolText.Text"=w188) -> ()  [unwired: 2 in, 2 out]
                n316 = property on="PC急停" class="Bool (严格)"("BoolText.Text"=w187) -> ()  [unwired: 2 in, 2 out]
                n317 = property on="PC正在换挡" class="Bool (严格)"("BoolText.Text"=w186) -> ()  [unwired: 2 in, 2 out]
                n318 = property on="PC换挡到位" class="Bool (严格)"("BoolText.Text"=w185) -> ()  [unwired: 2 in, 2 out]
                n319 = property on="PC换挡不成功" class="Bool (严格)"("BoolText.Text"=w184) -> ()  [unwired: 2 in, 2 out]
              }
              frame #4 {
                n320 = global read "全局 1.vi" "C-N设置"() -> (w197:string[])
                n321 = Index Array(array=w197) -> (element #1=w196:string, element #2=w195:string, element #3=w194:string, element #4=w193:string)  [unwired: 4 in]
                n322 = property on="设置" class="Str"("Text.Text"=w196) -> ()  [unwired: 2 in, 2 out]
                n323 = property on="退出" class="Bool"("BoolText.Text"=w195) -> ()  [unwired: 2 in, 2 out]
                n324 = property on="编辑配方" class="Bool"("BoolText.Text"=w194) -> ()  [unwired: 2 in, 2 out]
                n325 = property on="编辑设定参数" class="Bool"("BoolText.Text"=w193) -> ()  [unwired: 2 in, 2 out]
              }
              frame #5 {
                n326 = global read "全局 1.vi" "C-N目标档位"() -> (w200:string[])
                n327 = Index Array(array=w200) -> (element #1=w199:string, element #2=w198:string)  [unwired: 2 in]
                n328 = property on="UTACTOPC的目标档位" class="Str"("Text.Text"=w199) -> ()  [unwired: 2 in, 2 out]
                n329 = property on="档位目标" class="Str"("Text.Text"=w198) -> ()  [unwired: 2 in, 2 out]
              }
              frame #6 {
                n330 = global read "全局 1.vi" "C-N当前档位"() -> (w203:string[])
                n331 = Index Array(array=w203) -> (element #1=w202:string, element #2=w201:string)  [unwired: 2 in]
                n332 = property on="PCTOUTAC的当前档位" class="Str"("Text.Text"=w202) -> ()  [unwired: 2 in, 2 out]
                n333 = property on="当前档位" class="Str"("Text.Text"=w201) -> ()  [unwired: 2 in, 2 out]
              }
              frame #7 {
                n334 = global read "全局 1.vi" "C-N远程/本地"() -> (w206:string[])
                n335 = Index Array(array=w206) -> (element #1=w205:string, element #2=w204:string)  [unwired: 2 in]
                n336 = property on="远程/本地控制标题" class="Str"("Text.Text"=w205) -> ()  [unwired: 2 in, 2 out]
                n337 = property on="远程/本地控制" class="Bool (严格)"("BoolText.Text"=w204) -> ()  [unwired: 2 in, 2 out]
              }
            }
          }
          event "PC启动信号": Value Change {
            n338 = event-data() -> ()  [unwired: 1 in, 6 out]
            n339 = global write "全局 1.vi" "PCTOPLC发送启动信号"(TRUE ("PCTOPLC发送启动信号")) -> ()
          }
          event "擦除曲线": Value Change {
            # "初始化"
            n340 = event-data() -> ()  [unwired: 1 in, 6 out]
            n341 = call "初始化.vi"() -> ()  [unwired: 12 in]
          }
        }
      }
    }
  }
  n342 = And(x=w3, y=TRUE) -> (x .and. y?=w1:bool)
  n343 = UDP Close(connection ID=w5, 8:w4) -> ()  [unwired: 2 out]
  n344 = case shown="真" w1 {
    frame False {
    }
    frame True {
      n345 = invoke class="VI" method="FP.Close"() -> (reference out=w369:refnum<vi>, error out=w368:errorcluster)  [unwired: 3 in, 1 out]
      n346 = Close Reference(reference=w369, error in (no error)=w368) -> ()  [unwired: 1 out]
    }
  }
